vi "UMLEditor export.vi"(1 "graphics":refnum<class "Graphics.lvclass">, 2 "bounds":T1 {"height" format="%.2f"; "width" format="%.2f"; "y" format="%.2f"; "x" format="%.2f"}, 3 "exportype":T2, 4 "fileName":path, 5 "error in (no error)":errorcluster) -> (19 "error out":errorcluster)   [LabVIEW 2020]
doc: "Gets current diagram values"
uses:
  <resource>/Framework/Providers/Open_GDS/UML/UMLEditor/UMLEditor ExportType.ctl
  <resource>/Framework/Providers/Open_GDS/UML/Graphics_class/Graphics.lvclass
  <resource>/Framework/Providers/Open_GDS/UML/General/Rectangle/Rectangle Rectangle2D.ctl
panel:
  in  "Picture":picture
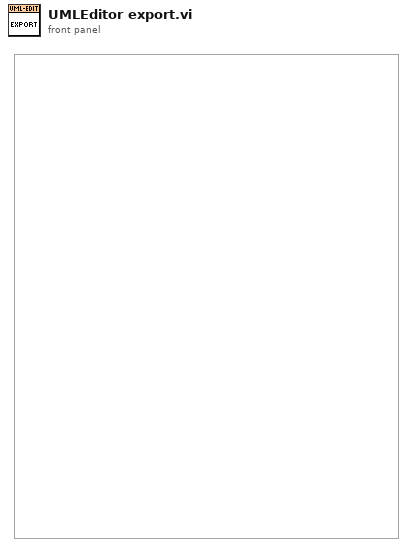
[diagram p1: front panel]
types:
  T1 = typedef "Rectangle Rectangle2D.ctl" = cluster{"x":dbl, "y":dbl, "width":dbl, "height":dbl}
  T2 = typedef "UMLEditor ExportType.ctl" = enum16{"None", "Printer", "png", "jpg", "roseUML"}
  T3 = cluster{"path":path, "orientation":u16, "PaperSize":i32, "PrinterName":string, "copies":i32}
  T4 = enum32{"existing file", "new file", "new or existing file", "existing dir", "new dir", "new or existing dir", "existing file (use LLBs)", "new file (use LLBs)", "new or existing file (use LLBs)", "new or existing file or directory (use LLBs)"}
  T5 = typedef "imagedata.ctl" = cluster{"image type":i32, "image depth":i32, "image":u8[], "mask":u8[], "colors":u32[], "Rectangle":cluster{"left":i16, "top":i16, "right":i16, "bottom":i16}}
  T6 = typedef "UMLEditor PrinterSettings.ctl" = cluster{"PrinterName":string, "Copies":i32, "PrintToFile":bool, "orientation":u16, "PaperSize":i32}
  T7 = typedef "LVRectTypeDef.ctl" = cluster{"left":i16, "top":i16, "right":i16, "bottom":i16}
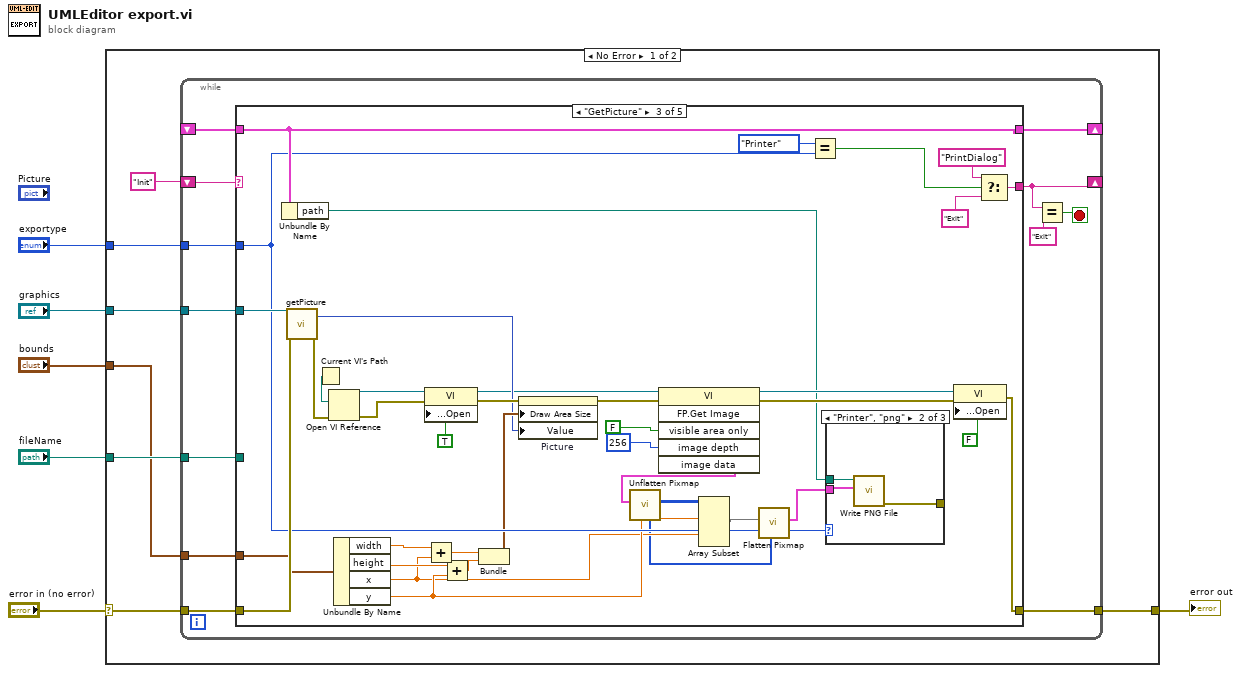
[diagram p0: block diagram]
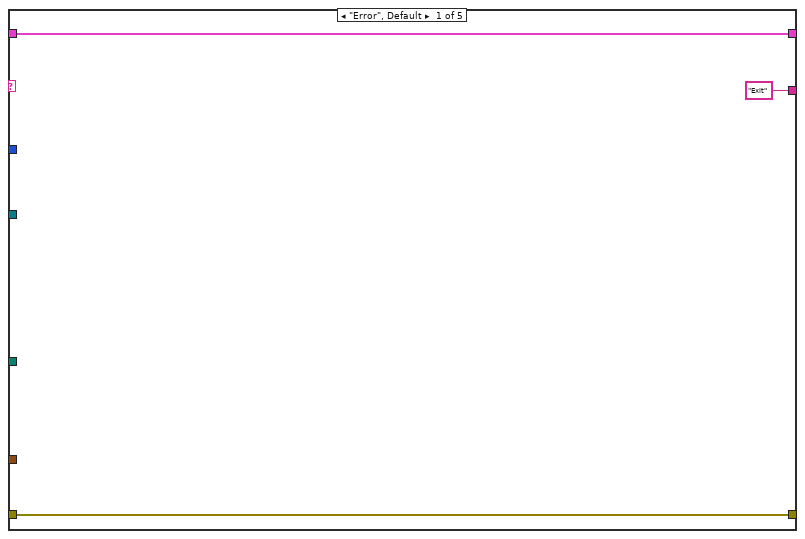
[diagram p2: hidden frame]
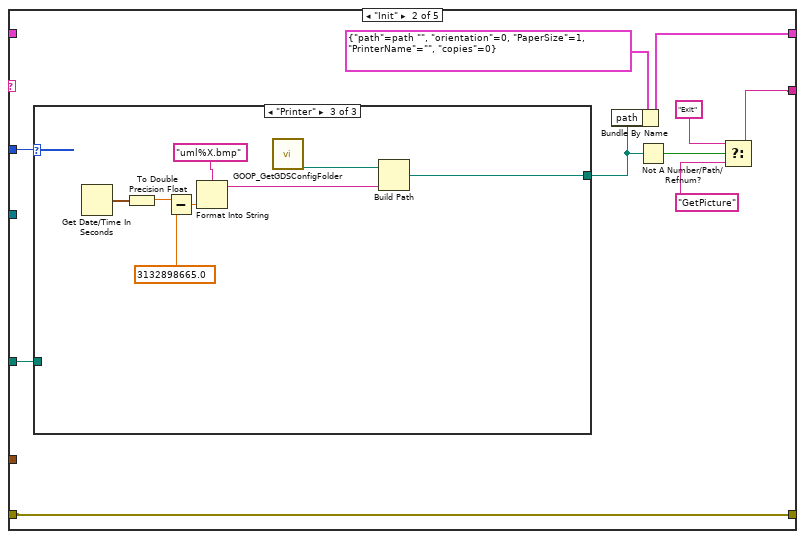
[diagram p3: hidden frame]
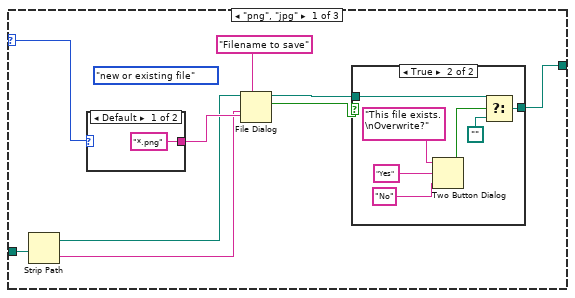
[diagram p4: hidden frame]
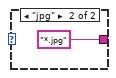
[diagram p6: hidden frame]
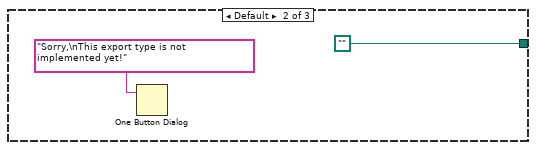
[diagram p7: hidden frame]
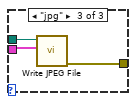
[diagram p9: hidden frame]
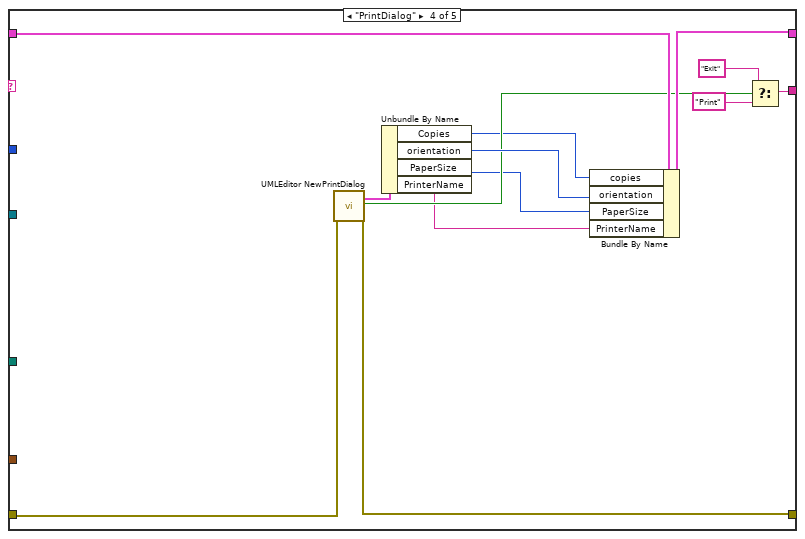
[diagram p10: hidden frame]
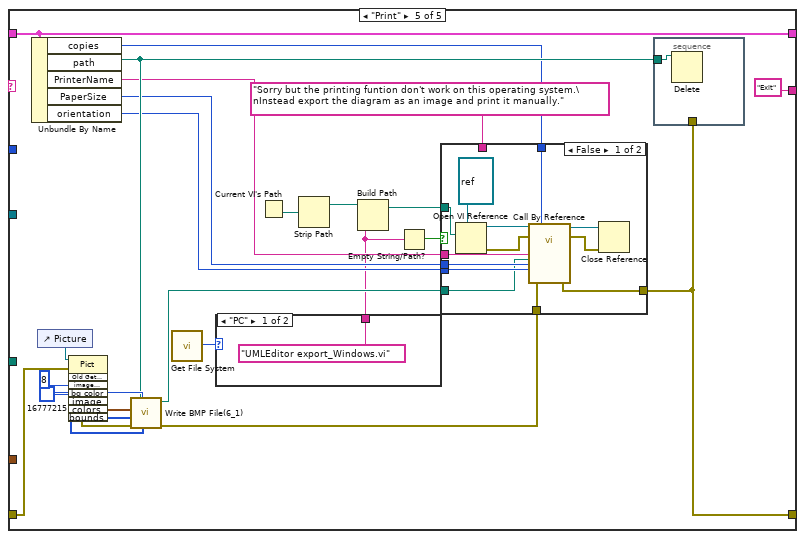
[diagram p11: hidden frame]
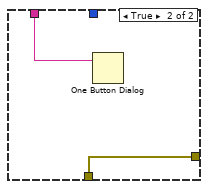
[diagram p12: hidden frame]
diagram:
  n1 = case shown="No Error" "error in (no error)" {
    selector: "error in (no error)" -> [w13 w167]
    tunnel: [w12 w167] -> w5
    tunnel: "fileName" -> [w8 _]
    tunnel: "graphics" -> [w11 _]
    tunnel: "exportype" -> [w9 _]
    tunnel: "bounds" -> [w7 _]
    frame No Error {
      n2 = while {
        tunnel: w13 -> [w25]
        tunnel: [w22] -> w12
        tunnel: w11 -> [w24]
        shift-right: [w21] -> _
        shift-left: "Init" -> [w23]
        shift-right: [w18] -> _
        shift-left: _ -> [w17]
        tunnel: w9 -> [w16]
        tunnel: w8 -> [w15]
        tunnel: w7 -> [w14]
        stop <- w19 stop-if-true
        n3 = case shown="\"GetPicture\"" w23 {
          tunnel: w25 -> [w28 w29 w105 w119 w139]
          tunnel: [w28 w29 w81 w118 w134] -> w22
          tunnel: w24 -> [_ _ w104 _ _]
          tunnel: ["Exit" w32 w98 w122 "Exit"] -> w21
          tunnel: [w26 w37 w95 w123 w148] -> w18
          tunnel: w17 -> [w26 _ w95 w124 w148]
          tunnel: w16 -> [_ w36 w88 _ _]
          tunnel: w15 -> [_ w30 _ _ _]
          tunnel: w14 -> [_ _ w85 _ _]
          frame "Error", Default {
          }
          frame "Init" {
            n4 = case shown="\"Printer\"" w36 {
              selector: w36 -> [w46 _ _]
              tunnel: [w43 path "" w64] -> w31
              tunnel: w30 -> [w41 _ _]
              frame "png", "jpg" {
                (unwired) T4."new or existing file" ("select mode (2)")
                n5 = Strip Path(path=w41) -> (stripped path=w40:path, name=w39:string)
                n6 = case shown="Default" w46 {
                  tunnel: ["*.png" ("pattern") "*.jpg" ("pattern")] -> w42
                  frame Default {
                  }
                  frame "jpg" {
                  }
                }
                n7 = File Dialog(6:w42, 7:"Filename to save" ("prompt"), 9:w39, 11:w40) -> (2:w45:bool, 3:w44:path)  [unwired: 1 in, 4 out]
                n8 = case shown="True" w45 {
                  tunnel: w44 -> [w48 w51]
                  tunnel: [w48 w50] -> w43
                  frame False {
                  }
                  frame True {
                    n9 = Two Button Dialog(message="This file exists.\nOverwrite?", 1:"No" ("F button name (\"Cancel\")"), 2:"Yes" ("T button name (\"OK\")")) -> (T button?=w52:bool)
                    n10 = Select(t=w51, s=w52, f=path "") -> (s? t:f=w50:path)
                  }
                }
              }
              frame Default {
                n11 = One Button Dialog(message="Sorry,\nThis export type is not implemented yet!") -> ()  [unwired: 2 out]
              }
              frame "Printer" {
                n12 = Get Date/Time In Seconds() -> (seconds since 1Jan1904=w60:timestamp)
                n13 = To Double Precision Float(number=w60) -> (double precision float=w62:dbl)
                n14 = Subtract(x=w62, y=3132898665.0 ("seconds since 1Jan1904")) -> (x-y=w63:dbl)
                n15 = Format Into String(format string="uml%X.bmp", w63) -> (resulting string=w66:string)  [unwired: 2 in, 1 out]
                n16 = call <resource>:"GOOP_GetGDSConfigFolder.vi"() -> ("GDSFolderPath"=w65:path)
                n17 = Build Path(base path=w65, name or relative path=w66) -> (appended path=w64:path)
              }
            }
            n18 = Bundle By Name(cluster=T3 {"path"=path "", "orientation"=0, "PaperSize"=1, "PrinterName"="", "copies"=0}, "path"=w31) -> (w37:T3)
            n19 = Not A Number/Path/Refnum?(number/path/refnum=w31) -> (NaN/Path/Refnum?=w35:bool)
            n20 = Select(t="Exit", s=w35, f="GetPicture") -> (s? t:f=w32:string)
          }
          frame "GetPicture" {
            n21 = Unbundle By Name(w95) -> ("path"=w89:path)
            n22 = call-dynamic "getPicture.vi"("reference"=w104, "error in (no error)"=w105) -> ("picture"=w83:picture, "error out"=w90:errorcluster)  [unwired: 16 out]
            n23 = Current VI's Path() -> (path=w94:path)
            n24 = Open VI Reference(vi path=w94, error in (no error)=w90) -> (vi reference=w79:refnum<vi>, error out=w80:errorcluster)  [unwired: 4 out]
            n25 = Unbundle By Name(w85) -> ("width"=w78:dbl, "height"=w76:dbl, "x"=w69:dbl, "y"=w70:dbl)
            n26 = property class="VI"(reference=w79, error in=w80, "Front Panel Window:Open"=TRUE) -> (reference out=w82:refnum<vi>, error out=w87:errorcluster)
            n27 = Add(x=w78, y=w69) -> (x+y=w77:dbl)
            n28 = Add(x=w76, y=w70) -> (x+y=w75:dbl)
            n29 = Bundle(w77, w75) -> (w84:cluster{dbl, dbl})  [unwired: 1 out]
            n30 = property on="Picture" class="Pict"(error in=w87, "Draw Area Size"=w84, "Value"=w83) -> (error out=w86:errorcluster)  [unwired: 1 in, 1 out]
            n31 = invoke class="VI" method="FP.Get Image"(reference=w82, error in=w86, "visible area only"=FALSE, "image depth"=256) -> (reference out=w103:refnum<vi>, error out=w102:errorcluster, "image data"=w72:T5)  [unwired: 2 in, 3 out]
            n32 = call <vilib>:"Unflatten Pixmap.vi"("image data"=w72) -> ("8-bit pixmap"=w74:u8[][], "colors"=w68:u32[])  [unwired: 4 in, 5 out]
            n33 = Array Subset(array=w74, index (row)=w70, index (col)=w69) -> (w73:u8[][])  [unwired: 2 in]
            n34 = call <vilib>:"Flatten Pixmap.vi"("colors"=w68, "8-bit pixmap"=w73) -> ("image data"=w71:T5)  [unwired: 9 in]
            n35 = Equal?(x=UMLEditor_ExportType."Printer", y=w88) -> (x = y?=w96:bool)
            n36 = case shown="\"Printer\", \"png\"" w88 {
              tunnel: w71 -> [_ w107 w110]
              tunnel: w89 -> [_ w108 w111]
              tunnel: [_ w106 w109] -> _
              frame Default {
              }
              frame "Printer", "png" {
                n37 = call <vilib>:"Write PNG File.vi"("image data"=w107, "path to PNG file"=w108) -> ("error out"=w106:errorcluster)  [unwired: 2 in, 7 out]
              }
              frame "jpg" {
                n38 = call <vilib>:"Write JPEG File.vi"("image data"=w110, "path to JPEG file"=w111) -> ("error out"=w109:errorcluster)  [unwired: 1 in, 8 out]
              }
            }
            n39 = property class="VI"(reference=w103, error in=w102, "Front Panel Window:Open"=FALSE) -> (error out=w81:errorcluster)  [unwired: 1 out]
            n40 = Select(t="PrintDialog", s=w96, f="Exit") -> (s? t:f=w98:string)
          }
          frame "PrintDialog" {
            n41 = call <resource>:"UMLEditor NewPrintDialog.vi"("error in (no error)"=w119) -> ("PrinterInfo"=w117:T6, "Cancelled"=w115:bool, "error out"=w118:errorcluster)  [unwired: 16 out]
            n42 = Unbundle By Name(w117) -> ("Copies"=w113:i32, "orientation"=w116:u16, "PaperSize"=w112:i32, "PrinterName"=w114:string)
            n43 = Bundle By Name(cluster=w124, "copies"=w113, "orientation"=w116, "PaperSize"=w112, "PrinterName"=w114) -> (w123:T3)
            n44 = Select(t="Exit", s=w115, f="Print") -> (s? t:f=w122:string)
          }
          frame "Print" {
            w146 = 8 ("image depth")
            n45 = Unbundle By Name(w148) -> ("copies"=w133:i32, "path"=w140:path, "PrinterName"=w138:string, "PaperSize"=w136:i32, "orientation"=w137:u16)
            n46 = control-ref of="Picture"() -> (w141:refnum<vi>)
            n47 = invoke class="Pict" method="Old Get Image"(reference=w141, error in=w139, "image depth"=w146, "bg color"=u32 16777215) -> (error out=w142:errorcluster, "image"=w143:u8[], "colors"=w144:u32[], "bounds"=w147:T7)  [unwired: 4 in, 4 out]
            n48 = call <vilib>:"Write BMP File(6_1).vi"("color table"=w144, "depth"=w146, "error in (no error)"=w142, "flattened image data"=w143, "rect"=w147, "path to BMP file"=w140) -> ("error out"=w135:errorcluster, "path"=w132:path)  [unwired: 4 out]
            n49 = call <vilib>:"Get File System.vi"() -> ("Platform (Unknown,Mac, Unix, PC)"=w130:enum16{"Unknown", "Mac", "Unix", "PC"})
            n50 = case shown="\"PC\"" w130 {
              tunnel: ["UMLEditor export_Windows.vi" _] -> w129
              frame "PC" {
              }
              frame Default {
              }
            }
            n51 = Current VI's Path() -> (path=w125:path)
            n52 = Strip Path(path=w125) -> (stripped path=w131:path)  [unwired: 1 out]
            n53 = Build Path(base path=w131, name or relative path=w129) -> (appended path=w126:path)
            n54 = Empty String/Path?(string/path=w129) -> (empty?=w128:bool)
            n55 = case shown="False" w128 {
              tunnel: w138 -> [w159 _]
              tunnel: w137 -> [w158 _]
              tunnel: w136 -> [w157 _]
              tunnel: w135 -> [w156 w164]
              tunnel: [w155 w164] -> w134
              tunnel: w133 -> [w154 _]
              tunnel: w132 -> [w151 _]
              tunnel: "Sorry but the printing funtion don't work on this operating system.\nInstead export the diagram as an image and print it manually." ("message") -> [_ w163]
              tunnel: w126 -> [w150 _]
              frame False {
                n56 = Open VI Reference(type specifier VI Refnum (for type only)=refnum<vi> refnum, vi path=w150) -> (vi reference=w160:refnum<vi>, error out=w161:errorcluster)  [unwired: 4 in]
                n57 = call-by-ref "?"(reference=w160, error in=w161, "PrinterName"=w159, "path"=w151, "PaperSize"=w157, "orientation"=w158, "error in"=w156, "copies"=w154) -> (reference out=w153:refnum<vi>, error out=w152:errorcluster, 19:"error out"=w155:errorcluster)  [unwired: 13 in]
                n58 = Close Reference(reference=w153, error in (no error)=w152) -> ()  [unwired: 1 out]
              }
              frame True {
                n59 = One Button Dialog(message=w163) -> ()  [unwired: 1 in, 1 out]
              }
            }
            n60 = stacked-sequence {
              tunnel: w140 -> [w166]
              tunnel: w134 -> [_]
              frame #0 {
                n61 = Delete(path (use dialog)=w166) -> ()  [unwired: 1 in, 6 out]
              }
            }
          }
        }
        n62 = Equal?(x=w21, y="Exit") -> (x = y?=w19:bool)
      }
    }
    frame Error {
    }
  }
  "error out" <- w5
